vi "TopVI_尬『電！阻』止這場災難吧！.vi"() -> ()   [LabVIEW 2014]
panel:
  in  "STORY":bool
  in  "HELP":bool
  in  "TIPS":bool
  in  "START":bool
  out "5th：":dbl format="%0.2f"
  out "4th：":dbl format="%0.2f"
  out "3rd：":dbl format="%0.2f"
  out "2nd :":dbl format="%0.2f"
  out "1st：":dbl format="%.2f"
  out "限時 !!":dbl=60.0 format="%0.2f"
  out "已答題數":i32
  out "Time":dbl format="%0.2f"
  out "錯誤次數":i32
  in  "QUIT":bool
  out "T_0":u32
  in  "Enter":bool
  out "Input 4":i32
  in  "Input 3":i32
  in  "Input 2":i32
  in  "Input 1":i32
  out "Color R4":u32(colorbox)
  out "Color R3":u32(colorbox)
  out "Color R2":u32(colorbox)
  out "Color R1":u32(colorbox)
  # "尬『電！阻』止這場災難吧！"
  # "É@Oo­^¶¯º]oOÉ@"
  # "(s)"
  # "(s)"
  # "(s)"
  # "(s)"
  # "x10   ±      % (Ω)"
  # "(s)"
  # "/ 5"
  # "/ 3"
  # "(s)"
  # "(s)"
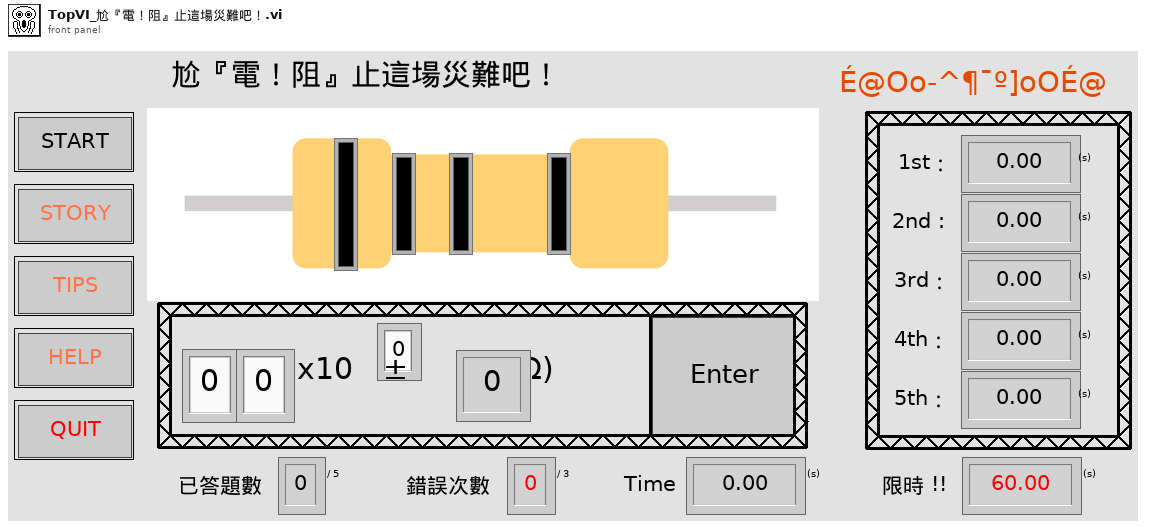
[diagram p1: front panel]
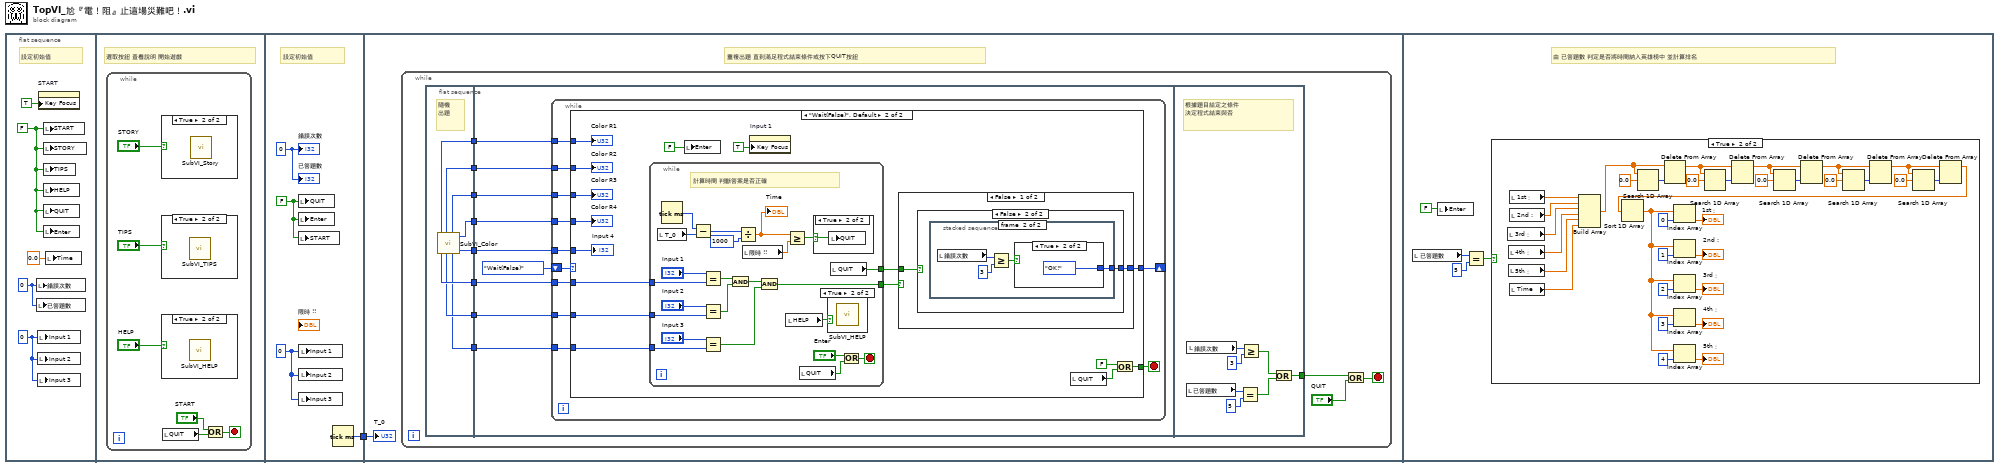
[diagram p0: block diagram]
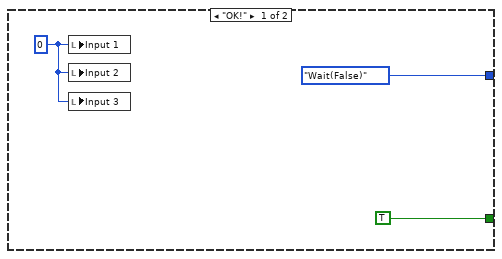
[diagram p5: hidden frame]
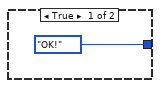
[diagram p8: hidden frame]
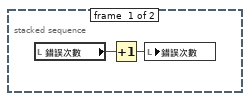
[diagram p9: hidden frame]
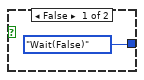
[diagram p10: hidden frame]
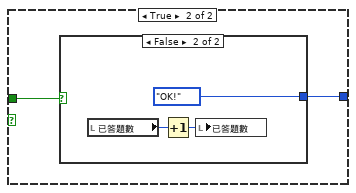
[diagram p11: hidden frame]
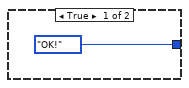
[diagram p12: hidden frame]
diagram:
  n1 = flat-sequence {
    tunnel: [w16] -> w1
    tunnel: w1 -> [w17]
    frame #0 {
      w2 = 0 ("Input 1")
      w3 = 0 ("錯誤次數")
      w4 = FALSE ("START")
      # "設定初始值"
      n2 = local write "錯誤次數"(w3) -> ()
      n3 = local write "已答題數"(w3) -> ()
      n4 = local write "Input 1"(w2) -> ()
      n5 = local write "Input 2"(w2) -> ()
      n6 = local write "Input 3"(w2) -> ()
      n7 = property on="START" class="Bool (strict)"("Key Focus"=TRUE) -> ()  [unwired: 2 in, 2 out]
      n8 = local write "START"(w4) -> ()
      n9 = local write "STORY"(w4) -> ()
      n10 = local write "TIPS"(w4) -> ()
      n11 = local write "HELP"(w4) -> ()
      n12 = local write "QUIT"(w4) -> ()
      n13 = local write "Enter"(w4) -> ()
      n14 = local write "Time"(0.0 ("Time")) -> ()
    }
    frame #1 {
      # "選取按鈕 查看說明 開始遊戲"
      n15 = while {
        stop <- w8 stop-if-true
        n16 = case shown="True" "STORY" {
          frame False {
          }
          frame True {
            n17 = call "SubVI_Story.vi"() -> ()  [unwired: 12 in]
          }
        }
        n18 = case shown="True" "TIPS" {
          frame False {
          }
          frame True {
            n19 = call "SubVI_TIPS.vi"() -> ()  [unwired: 12 in]
          }
        }
        n20 = case shown="True" "HELP" {
          frame False {
          }
          frame True {
            n21 = call "SubVI_HELP.vi"() -> ()  [unwired: 12 in]
          }
        }
        n22 = local read "QUIT"() -> (w9:bool)
        n23 = Or(x="START", y=w9) -> (x .or. y?=w8:bool)
      }
    }
    frame #2 {
      w14 = 0 ("Input 1")
      w13 = FALSE ("QUIT")
      w15 = 0 ("錯誤次數")
      # "設定初始值"
      n24 = local write "QUIT"(w13) -> ()
      n25 = local write "Enter"(w13) -> ()
      n26 = local write "START"(w13) -> ()
      n27 = local write "Input 1"(w14) -> ()
      n28 = local write "Input 2"(w14) -> ()
      n29 = local write "Input 3"(w14) -> ()
      n30 = Tick Count (ms)() -> (millisecond timer value=w16:u32)
      "錯誤次數" <- w15
      "已答題數" <- w15
    }
    frame #3 {
      # "重複出題 直到滿足程式結束條件或按下QUIT按鈕"
      n31 = while {
        stop <- w19 stop-if-true
        n32 = flat-sequence {
          tunnel: [w36] -> w28
          tunnel: [w35] -> w27
          tunnel: [w34] -> w26
          tunnel: [w33] -> w25
          tunnel: [w32] -> w24
          tunnel: [w31] -> w23
          tunnel: [w30] -> w22
          tunnel: [w29] -> w21
          tunnel: w28 -> [w45]
          tunnel: w27 -> [w44]
          tunnel: w26 -> [w43]
          tunnel: w25 -> [w42]
          tunnel: w24 -> [w41]
          tunnel: w23 -> [w40]
          tunnel: w22 -> [w39]
          tunnel: w21 -> [w38]
          tunnel: [w119] -> w18
          frame #0 {
            # "隨機\n出題"
            n33 = call "SubVI_Color.vi"() -> ("電阻值 1"=w36:u32, "電阻值 2"=w35:u32, "R1"=w31:i32, "R2"=w30:i32, "電阻值 3"=w34:u32, "電阻誤差"=w33:u32, "R3"=w29:i32, "R_error"=w32:i32)  [unwired: 2 in]
          }
          frame #1 {
            n34 = while {
              tunnel: w45 -> [w56]
              tunnel: w44 -> [w55]
              tunnel: w43 -> [w54]
              tunnel: w42 -> [w53]
              tunnel: w41 -> [w52]
              tunnel: w40 -> [w51]
              tunnel: w39 -> [w50]
              tunnel: w38 -> [w49]
              shift-right: [w47] -> _
              shift-left: enum16{"OK!", "Wait(False)"}."Wait(False)" -> [w48]
              stop <- w46 stop-if-true
              n35 = case shown="\"Wait(False)\", Default" w48 {
                tunnel: w56 -> [_ w74]
                tunnel: w55 -> [_ w73]
                tunnel: w54 -> [_ w72]
                tunnel: w53 -> [_ w71]
                tunnel: w52 -> [_ w70]
                tunnel: w51 -> [_ w66]
                tunnel: w50 -> [_ w65]
                tunnel: w49 -> [_ w64]
                tunnel: [enum16{"OK!", "Wait(False)"}."Wait(False)" w69] -> w47
                tunnel: [TRUE w63] -> w46
                frame "OK!" {
                  w57 = 0 ("Input 1")
                  n36 = local write "Input 1"(w57) -> ()
                  n37 = local write "Input 2"(w57) -> ()
                  n38 = local write "Input 3"(w57) -> ()
                }
                frame "Wait(False)", Default {
                  n39 = while {
                    tunnel: [w94] -> w67
                    tunnel: w66 -> [w93]
                    tunnel: w65 -> [w92]
                    tunnel: w64 -> [w91]
                    tunnel: [w77] -> w61
                    stop <- w83 stop-if-true
                    # "計算時間 判斷答案是否正確"
                    n40 = local read "T_0"() -> (w86:u32)
                    n41 = Tick Count (ms)() -> (millisecond timer value=w87:u32)
                    n42 = Subtract(x=w87, y=w86) -> (x-y=w85:u32)
                    n43 = Equal?(x="Input 1", y=w93) -> (x = y?=w98:bool)
                    n44 = Equal?(x="Input 2", y=w92) -> (x = y?=w97:bool)
                    n45 = Equal?(x="Input 3", y=w91) -> (x = y?=w95:bool)
                    n46 = And(x=w98, y=w97) -> (x .and. y?=w96:bool)
                    n47 = Divide(x=w85, y=u32 1000) -> (x/y=w80:dbl)
                    "Time" <- w80
                    n48 = local read "限時 !!"() -> (w79:dbl)
                    n49 = And(x=w96, y=w95) -> (x .and. y?=w94:bool)
                    n50 = local read "HELP"() -> (w76:bool)
                    n51 = Greater Or Equal?(x=w80, y=w79) -> (x >= y?=w78:bool)
                    n52 = local read "QUIT"() -> (w81:bool)
                    n53 = case shown="True" w78 {
                      selector: w78 -> [_ w99]
                      frame False {
                      }
                      frame True {
                        n54 = local write "QUIT"(w99) -> ()
                      }
                    }
                    n55 = case shown="True" w76 {
                      frame False {
                      }
                      frame True {
                        n56 = call "SubVI_HELP.vi"() -> ()  [unwired: 12 in]
                      }
                    }
                    n57 = local read "QUIT"() -> (w77:bool)
                    n58 = Or(x="Enter", y=w81) -> (x .or. y?=w83:bool)
                  }
                  n59 = local write "Enter"(FALSE ("Enter")) -> ()
                  n60 = property on="Input 1" class="DigNum (strict)"("Key Focus"=TRUE) -> ()  [unwired: 2 in, 2 out]
                  n61 = case shown="False" w67 {
                    tunnel: [w101 w113] -> w69
                    tunnel: w61 -> [w100 w112]
                    frame False {
                      n62 = case shown="False" w100 {
                        tunnel: [enum16{"OK!", "Wait(False)"}."OK!" w103] -> w101
                        frame True {
                        }
                        frame False {
                          n63 = stacked-sequence {
                            tunnel: [_ w109] -> w103
                            frame #0 {
                              n64 = local read "錯誤次數"() -> (w105:i32)
                              n65 = Increment(x=w105) -> (x+1=w104:i32)
                              n66 = local write "錯誤次數"(w104) -> ()
                            }
                            frame #1 {
                              n67 = local read "錯誤次數"() -> (w108:i32)
                              n68 = Greater Or Equal?(x=w108, y=3) -> (x >= y?=w106:bool)
                              n69 = case shown="True" w106 {
                                tunnel: [enum16{"OK!", "Wait(False)"}."Wait(False)" enum16{"OK!", "Wait(False)"}."OK!"] -> w109
                                frame False {
                                }
                                frame True {
                                }
                              }
                            }
                          }
                        }
                      }
                    }
                    frame True {
                      n70 = case shown="False" w112 {
                        tunnel: [enum16{"OK!", "Wait(False)"}."OK!" enum16{"OK!", "Wait(False)"}."OK!"] -> w113
                        frame True {
                        }
                        frame False {
                          n71 = local read "已答題數"() -> (w115:i32)
                          n72 = Increment(x=w115) -> (x+1=w116:i32)
                          n73 = local write "已答題數"(w116) -> ()
                        }
                      }
                    }
                  }
                  n74 = local read "QUIT"() -> (w60:bool)
                  n75 = Or(x=FALSE, y=w60) -> (x .or. y?=w63:bool)
                  "Color R1" <- w74
                  "Color R2" <- w73
                  "Color R3" <- w72
                  "Color R4" <- w71
                  "Input 4" <- w70
                }
              }
            }
          }
          frame #2 {
            # "根據題目給定之條件\n決定程式結束與否"
            n76 = local read "已答題數"() -> (w123:i32)
            n77 = local read "錯誤次數"() -> (w121:i32)
            n78 = Equal?(x=w123, y=5) -> (x = y?=w120:bool)
            n79 = Greater Or Equal?(x=w121, y=3) -> (x >= y?=w118:bool)
            n80 = Or(x=w118, y=w120) -> (x .or. y?=w119:bool)
          }
        }
        n81 = Or(x=w18, y="QUIT") -> (x .or. y?=w19:bool)
      }
      "T_0" <- w17
    }
    frame #4 {
      # "由 已答題數 判定是否將時間納入英雄榜中 並計算排名"
      n82 = local read "已答題數"() -> (w127:i32)
      n83 = local write "Enter"(FALSE ("Enter")) -> ()
      n84 = Equal?(x=w127, y=5) -> (x = y?=w126:bool)
      n85 = case shown="True" w126 {
        frame False {
        }
        frame True {
          n86 = local read "3rd："() -> (w159:dbl)
          n87 = local read "4th："() -> (w158:dbl)
          n88 = local read "5th："() -> (w157:dbl)
          n89 = local read "1st："() -> (w161:dbl)
          n90 = local read "2nd :"() -> (w160:dbl)
          n91 = local read "Time"() -> (w156:dbl)
          n92 = Build Array(w161, w160, w159, w158, w157, w156) -> (w141:dbl[])
          n93 = Search 1D Array(1D array=w141, element=0.0) -> (index of element=w142:i32)  [unwired: 1 in]
          n94 = Delete From Array(array=w141, index=w142) -> (array with subset deleted=w146:dbl[])  [unwired: 1 in, 1 out]
          n95 = Search 1D Array(1D array=w146, element=0.0) -> (index of element=w144:i32)  [unwired: 1 in]
          n96 = Delete From Array(array=w146, index=w144) -> (array with subset deleted=w149:dbl[])  [unwired: 1 in, 1 out]
          n97 = Search 1D Array(1D array=w149, element=0.0) -> (index of element=w147:i32)  [unwired: 1 in]
          n98 = Delete From Array(array=w149, index=w147) -> (array with subset deleted=w152:dbl[])  [unwired: 1 in, 1 out]
          n99 = Search 1D Array(1D array=w152, element=0.0) -> (index of element=w150:i32)  [unwired: 1 in]
          n100 = Delete From Array(array=w152, index=w150) -> (array with subset deleted=w155:dbl[])  [unwired: 1 in, 1 out]
          n101 = Search 1D Array(1D array=w155, element=0.0) -> (index of element=w153:i32)  [unwired: 1 in]
          n102 = Delete From Array(array=w155, index=w153) -> (array with subset deleted=w129:dbl[])  [unwired: 1 in, 1 out]
          n103 = Sort 1D Array(array=w129) -> (sorted array=w134:dbl[])
          n104 = Index Array(array=w134, index=0) -> (element=→"1st：":dbl)
          n105 = Index Array(array=w134, index=1) -> (element=→"2nd :":dbl)
          n106 = Index Array(array=w134, index=2) -> (element=→"3rd：":dbl)
          n107 = Index Array(array=w134, index=3) -> (element=→"4th：":dbl)
          n108 = Index Array(array=w134, index=4) -> (element=→"5th：":dbl)
        }
      }
    }
  }
